vi "HFRR ADV v017 new software.vi"() -> ()   [LabVIEW 2025] (continued)
            n2021 = String To Path(string=w2022) -> (path=w2030:path)
            n2022 = String To Path(string=w2021) -> (path=w2029:path)
            n2023 = String To Path(string=w2020) -> (path=w2028:path)
            n2024 = case shown="True" w2019 {
              tunnel: [w2035 w2036] -> w2023
              frame False {
                n2025 = local read "string1"() -> (w2035:string)
              }
              frame True {
                n2026 = local read "String Indicator 4"() -> (w2036:string)
              }
            }
            n2027 = Open/Create/Replace File "Open File"(file path (use dialog)=w2030) -> (refnum out=w2026:refnum<file>)  [unwired: 5 in, 2 out]
            n2028 = Open/Create/Replace File "Open File"(file path (use dialog)=w2029) -> (refnum out=w2025:refnum<file>)  [unwired: 5 in, 2 out]
            n2029 = Open/Create/Replace File "Open File"(file path (use dialog)=w2028) -> (refnum out=w2024:refnum<file>)  [unwired: 5 in, 2 out]
            n2030 = while {
              tunnel: w2026 -> [w2048]
              i -> [w2044]
              stop <- w2043 continue-if-true
              (unwired) TRUE ("line mode (F)")
              n2031 = Read from Text File "Read File"(file (use dialog)=w2048) -> (text=w2045:string)  [unwired: 3 in, 3 out]
              n2032 = local write "Numeric 11"(w2044) -> ()
              n2033 = String Length(string=w2045) -> (length=w2047:i32)
              n2034 = Greater?(x=w2047, y=1) -> (0:w2043:bool)
            }
            n2035 = while {
              tunnel: w2025 -> [w2054]
              i -> [w2050]
              stop <- w2049 continue-if-true
              (unwired) TRUE ("line mode (F)")
              n2036 = Read from Text File "Read File"(file (use dialog)=w2054) -> (text=w2051:string)  [unwired: 3 in, 3 out]
              n2037 = local write "Numeric 12"(w2050) -> ()
              n2038 = String Length(string=w2051) -> (length=w2053:i32)
              n2039 = Greater?(x=w2053, y=1) -> (0:w2049:bool)
            }
            n2040 = while {
              tunnel: w2024 -> [w2060]
              i -> [w2056]
              stop <- w2055 continue-if-true
              (unwired) TRUE ("line mode (F)")
              n2041 = Read from Text File "Read File"(file (use dialog)=w2060) -> (text=w2057:string)  [unwired: 3 in, 3 out]
              n2042 = local write "Numeric 13"(w2056) -> ()
              n2043 = String Length(string=w2057) -> (length=w2059:i32)
              n2044 = Greater?(x=w2059, y=1) -> (0:w2055:bool)
            }
            n2045 = String To Path(string=w2023) -> (path=w2031:path)
            n2046 = Open/Create/Replace File "Open File"(file path (use dialog)=w2031) -> (refnum out=w2027:refnum<file>)  [unwired: 5 in, 2 out]
            n2047 = while {
              tunnel: w2027 -> [w2042]
              i -> [w2038]
              stop <- w2037 continue-if-true
              (unwired) TRUE ("line mode (F)")
              n2048 = Read from Text File "Read File"(file (use dialog)=w2042) -> (text=w2039:string)  [unwired: 3 in, 3 out]
              n2049 = local write "Numeric 8"(w2038) -> ()
              n2050 = String Length(string=w2039) -> (length=w2041:i32)
              n2051 = Greater?(x=w2041, y=1) -> (0:w2037:bool)
            }
          }
          frame #1 {
            w2212 = FALSE ("ACTUAL   MERGE")
            # "Sample Temp"
            # "ECR"
            # "COF"
            # "Time\nCOF\nFF\nTemp"
            n2052 = case shown="True" w2085 {
              tunnel: [w2232 w2233] -> w2086
              frame False {
                n2053 = local read "string1"() -> (w2232:string)
              }
              frame True {
                n2054 = local read "String Indicator 4"() -> (w2233:string)
              }
            }
            n2055 = local read "string1 3"() -> (w2130:string)
            n2056 = String To Path(string=w2086) -> (path=w2217:path)
            n2057 = String To Path(string=w2130) -> (path=w2228:path)
            n2058 = local read "Numeric 12"() -> (w2214:i32)
            n2059 = local read "Numeric 8"() -> (w2216:i32)
            n2060 = local read "string1 2"() -> (w2131:string)
            n2061 = local read "string1 4"() -> (w2129:string)
            n2062 = Open/Create/Replace File "Open File"(file path (use dialog)=w2217) -> (refnum out=w2231:refnum<file>, error out=w2230:errorcluster)  [unwired: 5 in, 1 out]
            n2063 = Open/Create/Replace File "Open File"(file path (use dialog)=w2228) -> (refnum out=w2224:refnum<file>, error out=w2225:errorcluster)  [unwired: 5 in, 1 out]
            n2064 = for {
              N: w2216 -> [_]
              tunnel: w2231 -> [w2379]
              tunnel: w2230 -> [w2378]
              tunnel: [w2368] -> w2143 mode=indexing
              tunnel: [w2366] -> w2200 mode=indexing
              tunnel: [w2367] -> w2195 mode=indexing
              tunnel: w2212 -> [_]
              tunnel: [w2360] -> w2197 mode=indexing
              tunnel: [w2356] -> w2166 mode=indexing
              tunnel: [w2352] -> w2141 mode=indexing
              tunnel: [w2348] -> w2122 mode=indexing
              tunnel: [w2343] -> w2082 mode=indexing
              (unwired) TRUE ("line mode (F)")
              # "freq"
              # "Stroke"
              # "Time"
              # "CoF"
              # "Humidity"
              # "Temp"
              # "Air Temp"
              # "ECR"
              n2065 = Read from Text File "Read File"(file (use dialog)=w2379, error in=w2378) -> (text=w2344:string)  [unwired: 2 in, 3 out]
              n2066 = local write "String 6"(w2344) -> ()
              n2067 = String Subset(string=w2344, offset (0)=0, length (rest)=14 ("length (rest)")) -> (substring=w2372:string)
              n2068 = String Subset(string=w2344, offset (0)=35, length (rest)=9 ("length (rest)")) -> (substring=w2369:string)
              n2069 = String Subset(string=w2344, offset (0)=15, length (rest)=9 ("length (rest)")) -> (substring=w2375:string)
              n2070 = Fract/Exp String To Number(string=w2372) -> (number=w2368:dbl)  [unwired: 3 in, 1 out]
              n2071 = Fract/Exp String To Number(string=w2369) -> (number=w2367:dbl)  [unwired: 3 in, 1 out]
              n2072 = Fract/Exp String To Number(string=w2375) -> (number=w2366:dbl)  [unwired: 3 in, 1 out]
              n2073 = String Subset(string=w2344, offset (0)=85, length (rest)=9 ("length (rest)")) -> (substring=w2345:string)
              n2074 = String Subset(string=w2344, offset (0)=25, length (rest)=9 ("length (rest)")) -> (substring=w2351:string)
              n2075 = String Subset(string=w2344, offset (0)=55, length (rest)=9 ("length (rest)")) -> (substring=w2353:string)
              n2076 = String Subset(string=w2344, offset (0)=45, length (rest)=9 ("length (rest)")) -> (substring=w2359:string)
              n2077 = String Subset(string=w2344, offset (0)=65, length (rest)=9 ("length (rest)")) -> (substring=w2365:string)
              n2078 = Fract/Exp String To Number(string=w2351) -> (number=w2348:dbl)  [unwired: 3 in, 1 out]
              n2079 = Fract/Exp String To Number(string=w2345) -> (number=w2343:dbl)  [unwired: 3 in, 1 out]
              n2080 = Fract/Exp String To Number(string=w2353) -> (number=w2352:dbl)  [unwired: 3 in, 1 out]
              n2081 = Fract/Exp String To Number(string=w2359) -> (number=w2356:dbl)  [unwired: 3 in, 1 out]
              n2082 = Fract/Exp String To Number(string=w2365) -> (number=w2362:dbl)  [unwired: 3 in, 1 out]
              n2083 = Add(x=w2362, y=0.0) -> (x+y=w2360:dbl)
            }
            n2084 = for {
              N: w2214 -> [_]
              tunnel: w2225 -> [w2305]
              tunnel: w2224 -> [w2304]
              tunnel: [w2294] -> w2183 mode=indexing
              tunnel: [w2292] -> w2181 mode=indexing
              tunnel: [w2293] -> w2177 mode=indexing
              tunnel: w2212 -> [_]
              tunnel: [w2286] -> w2179 mode=indexing
              tunnel: [w2282] -> w2161 mode=indexing
              tunnel: [w2278] -> w2137 mode=indexing
              tunnel: [w2275] -> w2118 mode=indexing
              tunnel: [w2271] -> w2077 mode=indexing
              (unwired) 9 ("length (rest)")
              (unwired) 9 ("length (rest)")
              (unwired) TRUE ("line mode (F)")
              n2085 = Read from Text File "Read File"(file (use dialog)=w2304, error in=w2305) -> (text=w2272:string)  [unwired: 2 in, 3 out]
              n2086 = local write "String 8"(w2272) -> ()
              n2087 = String Subset(string=w2272, offset (0)=85) -> (substring=w2274:string)  [unwired: 1 in]
              n2088 = String Subset(string=w2272, offset (0)=35, length (rest)=9 ("length (rest)")) -> (substring=w2295:string)
              n2089 = String Subset(string=w2272, offset (0)=55, length (rest)=9 ("length (rest)")) -> (substring=w2280:string)
              n2090 = String Subset(string=w2272, offset (0)=25) -> (substring=w2276:string)  [unwired: 1 in]
              n2091 = String Subset(string=w2272, offset (0)=15, length (rest)=9 ("length (rest)")) -> (substring=w2301:string)
              n2092 = String Subset(string=w2272, offset (0)=0, length (rest)=14 ("length (rest)")) -> (substring=w2298:string)
              n2093 = String Subset(string=w2272, offset (0)=45, length (rest)=9 ("length (rest)")) -> (substring=w2285:string)
              n2094 = String Subset(string=w2272, offset (0)=65, length (rest)=9 ("length (rest)")) -> (substring=w2291:string)
              n2095 = Fract/Exp String To Number(string=w2274) -> (number=w2271:dbl)  [unwired: 3 in, 1 out]
              n2096 = Fract/Exp String To Number(string=w2295) -> (number=w2293:dbl)  [unwired: 3 in, 1 out]
              n2097 = Fract/Exp String To Number(string=w2280) -> (number=w2278:dbl)  [unwired: 3 in, 1 out]
              n2098 = Fract/Exp String To Number(string=w2276) -> (number=w2275:dbl)  [unwired: 3 in, 1 out]
              n2099 = Fract/Exp String To Number(string=w2301) -> (number=w2292:dbl)  [unwired: 3 in, 1 out]
              n2100 = Fract/Exp String To Number(string=w2298) -> (number=w2294:dbl)  [unwired: 3 in, 1 out]
              n2101 = Fract/Exp String To Number(string=w2285) -> (number=w2282:dbl)  [unwired: 3 in, 1 out]
              n2102 = Fract/Exp String To Number(string=w2291) -> (number=w2288:dbl)  [unwired: 3 in, 1 out]
              n2103 = Add(x=w2288, y=0.0) -> (x+y=w2286:dbl)
            }
            n2104 = String To Path(string=w2131) -> (path=w2229:path)
            n2105 = String To Path(string=w2129) -> (path=w2223:path)
            n2106 = local read "Numeric 11"() -> (w2213:i32)
            n2107 = local read "Numeric 13"() -> (w2215:i32)
            n2108 = Open/Create/Replace File "Open File"(file path (use dialog)=w2229) -> (refnum out=w2227:refnum<file>, error out=w2226:errorcluster)  [unwired: 5 in, 1 out]
            n2109 = Open/Create/Replace File "Open File"(file path (use dialog)=w2223) -> (refnum out=w2222:refnum<file>, error out=w2221:errorcluster)  [unwired: 5 in, 1 out]
            n2110 = for {
              N: w2213 -> [_]
              tunnel: w2227 -> [w2342]
              tunnel: w2226 -> [w2341]
              tunnel: [w2331] -> w2193 mode=indexing
              tunnel: [w2329] -> w2191 mode=indexing
              tunnel: [w2330] -> w2186 mode=indexing
              tunnel: w2212 -> [_]
              tunnel: [w2323] -> w2188 mode=indexing
              tunnel: [w2319] -> w2164 mode=indexing
              tunnel: [w2315] -> w2139 mode=indexing
              tunnel: [w2311] -> w2120 mode=indexing
              tunnel: [w2306] -> w2078 mode=indexing
              (unwired) TRUE ("line mode (F)")
              n2111 = Read from Text File "Read File"(file (use dialog)=w2342, error in=w2341) -> (text=w2307:string)  [unwired: 2 in, 3 out]
              n2112 = local write "String 7"(w2307) -> ()
              n2113 = String Subset(string=w2307, offset (0)=85, length (rest)=9 ("length (rest)")) -> (substring=w2310:string)
              n2114 = String Subset(string=w2307, offset (0)=35, length (rest)=9 ("length (rest)")) -> (substring=w2332:string)
              n2115 = String Subset(string=w2307, offset (0)=55, length (rest)=9 ("length (rest)")) -> (substring=w2318:string)
              n2116 = String Subset(string=w2307, offset (0)=25, length (rest)=9 ("length (rest)")) -> (substring=w2312:string)
              n2117 = String Subset(string=w2307, offset (0)=45, length (rest)=9 ("length (rest)")) -> (substring=w2320:string)
              n2118 = String Subset(string=w2307, offset (0)=0, length (rest)=14 ("length (rest)")) -> (substring=w2335:string)
              n2119 = String Subset(string=w2307, offset (0)=15, length (rest)=9 ("length (rest)")) -> (substring=w2338:string)
              n2120 = String Subset(string=w2307, offset (0)=65, length (rest)=9 ("length (rest)")) -> (substring=w2324:string)
              n2121 = Fract/Exp String To Number(string=w2310) -> (number=w2306:dbl)  [unwired: 3 in, 1 out]
              n2122 = Fract/Exp String To Number(string=w2332) -> (number=w2330:dbl)  [unwired: 3 in, 1 out]
              n2123 = Fract/Exp String To Number(string=w2318) -> (number=w2315:dbl)  [unwired: 3 in, 1 out]
              n2124 = Fract/Exp String To Number(string=w2312) -> (number=w2311:dbl)  [unwired: 3 in, 1 out]
              n2125 = Fract/Exp String To Number(string=w2320) -> (number=w2319:dbl)  [unwired: 3 in, 1 out]
              n2126 = Fract/Exp String To Number(string=w2335) -> (number=w2331:dbl)  [unwired: 3 in, 1 out]
              n2127 = Fract/Exp String To Number(string=w2338) -> (number=w2329:dbl)  [unwired: 3 in, 1 out]
              n2128 = Fract/Exp String To Number(string=w2324) -> (number=w2327:dbl)  [unwired: 3 in, 1 out]
              n2129 = Add(x=w2327, y=0.0) -> (x+y=w2323:dbl)
            }
            n2130 = for {
              N: w2215 -> [_]
              tunnel: w2222 -> [w2270]
              tunnel: w2221 -> [w2269]
              tunnel: [w2259] -> w2175 mode=indexing
              tunnel: [w2258] -> w2168 mode=indexing
              tunnel: w2212 -> [_]
              tunnel: [w2247] -> w2173 mode=indexing
              tunnel: [w2252] -> w2170 mode=indexing
              tunnel: [w2248] -> w2160 mode=indexing
              tunnel: [w2243] -> w2135 mode=indexing
              tunnel: [w2239] -> w2116 mode=indexing
              tunnel: [w2234] -> w2076 mode=indexing
              (unwired) 1.0 ("x")
              (unwired) TRUE ("line mode (F)")
              n2131 = Read from Text File "Read File"(file (use dialog)=w2270, error in=w2269) -> (text=w2235:string)  [unwired: 2 in, 3 out]
              n2132 = local write "String 12"(w2235) -> ()
              n2133 = String Subset(string=w2235, offset (0)=85, length (rest)=9 ("length (rest)")) -> (substring=w2237:string)
              n2134 = String Subset(string=w2235, offset (0)=35, length (rest)=9 ("length (rest)")) -> (substring=w2260:string)
              n2135 = String Subset(string=w2235, offset (0)=55, length (rest)=9 ("length (rest)")) -> (substring=w2245:string)
              n2136 = String Subset(string=w2235, offset (0)=25, length (rest)=9 ("length (rest)")) -> (substring=w2241:string)
              n2137 = String Subset(string=w2235, offset (0)=45, length (rest)=9 ("length (rest)")) -> (substring=w2250:string)
              n2138 = String Subset(string=w2235, offset (0)=15, length (rest)=9 ("length (rest)")) -> (substring=w2266:string)
              n2139 = String Subset(string=w2235, offset (0)=0, length (rest)=14 ("length (rest)")) -> (substring=w2263:string)
              n2140 = String Subset(string=w2235, offset (0)=65, length (rest)=9 ("length (rest)")) -> (substring=w2253:string)
              n2141 = Fract/Exp String To Number(string=w2237) -> (number=w2234:dbl)  [unwired: 3 in, 1 out]
              n2142 = Fract/Exp String To Number(string=w2260) -> (number=w2258:dbl)  [unwired: 3 in, 1 out]
              n2143 = Fract/Exp String To Number(string=w2245) -> (number=w2243:dbl)  [unwired: 3 in, 1 out]
              n2144 = Fract/Exp String To Number(string=w2241) -> (number=w2239:dbl)  [unwired: 3 in, 1 out]
              n2145 = Fract/Exp String To Number(string=w2250) -> (number=w2248:dbl)  [unwired: 3 in, 1 out]
              n2146 = Fract/Exp String To Number(string=w2266) -> (number=w2247:dbl)  [unwired: 3 in, 1 out]
              n2147 = Fract/Exp String To Number(string=w2263) -> (number=w2259:dbl)  [unwired: 3 in, 1 out]
              n2148 = Fract/Exp String To Number(string=w2253) -> (number=w2256:dbl)  [unwired: 3 in, 1 out]
              n2149 = Add(x=w2256, y=0.0) -> (x+y=w2252:dbl)
            }
            n2150 = Delete From Array(array=w2118, index=0) -> (array with subset deleted=w2091:dbl[])  [unwired: 1 in, 1 out]
            n2151 = Delete From Array(array=w2181, index=0) -> (array with subset deleted=w2154:dbl[])  [unwired: 1 in, 1 out]
            n2152 = Delete From Array(array=w2161, index=0) -> (array with subset deleted=w2149:dbl[])  [unwired: 1 in, 1 out]
            n2153 = Delete From Array(array=w2179, index=0) -> (array with subset deleted=w2180:dbl[])  [unwired: 1 in, 1 out]
            n2154 = call-poly <vilib>:"Mean.vi"("X"=w2091) -> ("mean"=→"КОФ2 4":dbl)  [unwired: 1 out]
            n2155 = call-poly <vilib>:"Mean.vi"("X"=w2154) -> ("mean"=→"КОФ3":dbl)  [unwired: 1 out]
            n2156 = call-poly <vilib>:"Mean.vi"("X"=w2149) -> ("mean"=→"CP3":dbl)  [unwired: 1 out]
            n2157 = Delete From Array(array=w2143, index=0) -> (array with subset deleted=w2070:dbl[])  [unwired: 1 in, 1 out]
            n2158 = Delete From Array(array=w2082, index=0) -> (array with subset deleted=w2069:dbl[])  [unwired: 1 in, 1 out]
            n2159 = Delete From Array(array=w2122, index=0) -> (array with subset deleted=w2093:dbl[])  [unwired: 1 in, 1 out]
            n2160 = Delete From Array(array=w2200, index=0) -> (array with subset deleted=w2155:dbl[])  [unwired: 1 in, 1 out]
            n2161 = Delete From Array(array=w2166, index=0) -> (array with subset deleted=w2151:dbl[])  [unwired: 1 in, 1 out]
            "array w/ subset deleted" <- w2151
            n2162 = Delete From Array(array=w2197, index=0) -> (array with subset deleted=w2198:dbl[])  [unwired: 1 in, 1 out]
            n2163 = call-poly <vilib>:"Mean.vi"("X"=w2093) -> ("mean"=→"КОФ2 2":dbl)  [unwired: 1 out]
            n2164 = call-poly <vilib>:"Mean.vi"("X"=w2155) -> ("mean"=→"КОФ1":dbl)  [unwired: 1 out]
            n2165 = Bundle "Bundle"(w2070, w2069) -> (w2075:cluster{dbl[], dbl[]})  [unwired: 1 in]
            n2166 = Bundle "Bundle"(w2070, w2198) -> (w2062:cluster{dbl[], dbl[]})  [unwired: 1 in]
            n2167 = Delete From Array(array=w2077, index=0) -> (array with subset deleted=w2065:dbl[])  [unwired: 1 in, 1 out]
            n2168 = Delete From Array(array=w2078, index=0) -> (array with subset deleted=w2067:dbl[])  [unwired: 1 in, 1 out]
            n2169 = Delete From Array(array=w2188, index=0) -> (array with subset deleted=w2189:dbl[])  [unwired: 1 in, 1 out]
            n2170 = Delete From Array(array=w2076, index=0) -> (array with subset deleted=w2063:dbl[])  [unwired: 1 in, 1 out]
            n2171 = Delete From Array(array=w2170, index=0) -> (array with subset deleted=w2171:dbl[])  [unwired: 1 in, 1 out]
            n2172 = Delete From Array(array=w2195, index=0) -> (array with subset deleted=w2101:dbl[])  [unwired: 1 in, 1 out]
            n2173 = Delete From Array(array=w2141, index=0) -> (array with subset deleted=w2097:dbl[])  [unwired: 1 in, 1 out]
            n2174 = Delete From Array(array=w2177, index=0) -> (array with subset deleted=w2099:dbl[])  [unwired: 1 in, 1 out]
            n2175 = Delete From Array(array=w2137, index=0) -> (array with subset deleted=w2095:dbl[])  [unwired: 1 in, 1 out]
            n2176 = Delete From Array(array=w2186, index=0) -> (array with subset deleted=w2100:dbl[])  [unwired: 1 in, 1 out]
            n2177 = Delete From Array(array=w2139, index=0) -> (array with subset deleted=w2096:dbl[])  [unwired: 1 in, 1 out]
            n2178 = Delete From Array(array=w2120, index=0) -> (array with subset deleted=w2092:dbl[])  [unwired: 1 in, 1 out]
            n2179 = Delete From Array(array=w2164, index=0) -> (array with subset deleted=w2150:dbl[])  [unwired: 1 in, 1 out]
            n2180 = Delete From Array(array=w2191, index=0) -> (array with subset deleted=w2152:dbl[])  [unwired: 1 in, 1 out]
            n2181 = Delete From Array(array=w2168, index=0) -> (array with subset deleted=w2098:dbl[])  [unwired: 1 in, 1 out]
            n2182 = Delete From Array(array=w2135, index=0) -> (array with subset deleted=w2094:dbl[])  [unwired: 1 in, 1 out]
            n2183 = Delete From Array(array=w2116, index=0) -> (array with subset deleted=w2090:dbl[])  [unwired: 1 in, 1 out]
            n2184 = Delete From Array(array=w2160, index=0) -> (array with subset deleted=w2148:dbl[])  [unwired: 1 in, 1 out]
            n2185 = Delete From Array(array=w2173, index=0) -> (array with subset deleted=w2153:dbl[])  [unwired: 1 in, 1 out]
            n2186 = Delete From Array(array=w2183, index=0) -> (array with subset deleted=w2066:dbl[])  [unwired: 1 in, 1 out]
            n2187 = Delete From Array(array=w2193, index=0) -> (array with subset deleted=w2068:dbl[])  [unwired: 1 in, 1 out]
            n2188 = Delete From Array(array=w2175, index=0) -> (array with subset deleted=w2064:dbl[])  [unwired: 1 in, 1 out]
            n2189 = Bundle "Bundle"(w2070, w2101) -> (w2088:cluster{dbl[], dbl[]})  [unwired: 1 in]
            n2190 = Bundle "Bundle"(w2070, w2155) -> (w2089:cluster{dbl[], dbl[]})  [unwired: 1 in]
            n2191 = Bundle "Bundle"(w2101, w2097) -> (w2103:cluster{dbl[], dbl[]})  [unwired: 1 in]
            n2192 = Bundle "Bundle"(w2066, w2065) -> (w2073:cluster{dbl[], dbl[]})  [unwired: 1 in]
            n2193 = Bundle "Bundle"(w2099, w2095) -> (w2105:cluster{dbl[], dbl[]})  [unwired: 1 in]
            n2194 = Bundle "Bundle"(w2066, w2099) -> (w2209:cluster{dbl[], dbl[]})  [unwired: 1 in]
            n2195 = Bundle "Bundle"(w2066, w2095) -> (w2133:cluster{dbl[], dbl[]})  [unwired: 1 in]
            n2196 = Bundle "Bundle"(w2066, w2154) -> (w2219:cluster{dbl[], dbl[]})  [unwired: 1 in]
            n2197 = Bundle "Bundle"(w2066, w2149) -> (w2157:cluster{dbl[], dbl[]})  [unwired: 1 in]
            n2198 = Bundle "Bundle"(w2066, w2180) -> (w2204:cluster{dbl[], dbl[]})  [unwired: 1 in]
            n2199 = Bundle "Bundle"(w2100, w2096) -> (w2104:cluster{dbl[], dbl[]})  [unwired: 1 in]
            n2200 = Bundle "Bundle"(w2068, w2067) -> (w2074:cluster{dbl[], dbl[]})  [unwired: 1 in]
            n2201 = Bundle "Bundle"(w2068, w2100) -> (w2211:cluster{dbl[], dbl[]})  [unwired: 1 in]
            n2202 = Bundle "Bundle"(w2068, w2096) -> (w2134:cluster{dbl[], dbl[]})  [unwired: 1 in]
            n2203 = Bundle "Bundle"(w2068, w2150) -> (w2158:cluster{dbl[], dbl[]})  [unwired: 1 in]
            n2204 = Bundle "Bundle"(w2068, w2152) -> (w2220:cluster{dbl[], dbl[]})  [unwired: 1 in]
            n2205 = Bundle "Bundle"(w2068, w2189) -> (w2202:cluster{dbl[], dbl[]})  [unwired: 1 in]
            n2206 = Bundle "Bundle"(w2098, w2094) -> (w2106:cluster{dbl[], dbl[]})  [unwired: 1 in]
            n2207 = Bundle "Bundle"(w2064, w2063) -> (w2072:cluster{dbl[], dbl[]})  [unwired: 1 in]
            n2208 = Bundle "Bundle"(w2064, w2098) -> (w2210:cluster{dbl[], dbl[]})  [unwired: 1 in]
            n2209 = Bundle "Bundle"(w2064, w2094) -> (w2132:cluster{dbl[], dbl[]})  [unwired: 1 in]
            n2210 = Bundle "Bundle"(w2064, w2148) -> (w2156:cluster{dbl[], dbl[]})  [unwired: 1 in]
            n2211 = Bundle "Bundle"(w2064, w2153) -> (w2218:cluster{dbl[], dbl[]})  [unwired: 1 in]
            n2212 = Bundle "Bundle"(w2064, w2171) -> (w2203:cluster{dbl[], dbl[]})  [unwired: 1 in]
            n2213 = call-poly <vilib>:"Mean.vi"("X"=w2151) -> ("mean"=→"CP1":dbl)  [unwired: 1 out]
            n2214 = call-poly <vilib>:"Mean.vi"("X"=w2092) -> ("mean"=→"КОФ2 3":dbl)  [unwired: 1 out]
            n2215 = call-poly <vilib>:"Mean.vi"("X"=w2150) -> ("mean"=→"CP2":dbl)  [unwired: 1 out]
            n2216 = call-poly <vilib>:"Mean.vi"("X"=w2152) -> ("mean"=→"КОФ2":dbl)  [unwired: 1 out]
            n2217 = call-poly <vilib>:"Mean.vi"("X"=w2090) -> ("mean"=→"КОФ2 5":dbl)  [unwired: 1 out]
            n2218 = call-poly <vilib>:"Mean.vi"("X"=w2148) -> ("mean"=→"CP4":dbl)  [unwired: 1 out]
            n2219 = call-poly <vilib>:"Mean.vi"("X"=w2153) -> ("mean"=→"КОФ4":dbl)  [unwired: 1 out]
            n2220 = Bundle "Bundle"(w2070, w2097) -> (w2061:cluster{dbl[], dbl[]})  [unwired: 1 in]
            n2221 = Bundle "Bundle"(w2070, w2151) -> (w2084:cluster{dbl[], dbl[]})  [unwired: 1 in]
            n2222 = Build Array "Build Array"(w2061, w2084) -> (w2087:cluster{dbl[], dbl[]}[])
            "XY Graph 17" <- w2087
            n2223 = Build Array "Build Array"(w2075, w2074, w2073, w2072) -> (→"Frequency ( Hz )":cluster{dbl[], dbl[]}[])
            n2224 = Build Array "Build Array"(w2103, w2104, w2105, w2106) -> (→"Air Temp ( °C ) vs Humidity ( % RH )":cluster{dbl[], dbl[]}[])
            n2225 = Build Array "Build Array"(w2088, w2211, w2209, w2210) -> (→"Air Temperature  ( °C )":cluster{dbl[], dbl[]}[])
            n2226 = Build Array "Build Array"(w2061, w2134, w2133, w2132) -> (→"Humidity ( %RH )":cluster{dbl[], dbl[]}[])
            n2227 = Build Array "Build Array"(w2089, w2220, w2219, w2218) -> (→"Coefficient Of Friction":cluster{dbl[], dbl[]}[])
            n2228 = Build Array "Build Array"(w2084, w2158, w2157, w2156) -> (→"Sample Temperature ( °C )":cluster{dbl[], dbl[]}[])
            n2229 = Build Array "Build Array"(w2062, w2202, w2204, w2203) -> (→"XY Graph 13":cluster{dbl[], dbl[]}[])
            n2230 = Bundle "Bundle"(w2070, w2093) -> (w2115:cluster{dbl[], dbl[]})  [unwired: 1 in]
            n2231 = Bundle "Bundle"(w2066, w2091) -> (w2113:cluster{dbl[], dbl[]})  [unwired: 1 in]
            n2232 = Bundle "Bundle"(w2068, w2092) -> (w2114:cluster{dbl[], dbl[]})  [unwired: 1 in]
            n2233 = Bundle "Bundle"(w2064, w2090) -> (w2112:cluster{dbl[], dbl[]})  [unwired: 1 in]
            n2234 = Build Array "Build Array"(w2115, w2114, w2113, w2112) -> (→"Stroke ( mm )":cluster{dbl[], dbl[]}[])
            n2235 = local write "XY Graph 16"(w2087) -> ()
          }
          frame #2 {
          }
          frame #3 {
            n2236 = local write "Numeric 8"(0 ("Numeric 8")) -> ()
            n2237 = local write "Numeric 11"(0 ("Numeric 11")) -> ()
            n2238 = local write "Numeric 12"(0 ("Numeric 12")) -> ()
            n2239 = local write "Numeric 13"(0 ("Numeric 13")) -> ()
            n2240 = property on="OPEN" class="Bool (strict)"("Visible"=TRUE) -> ()  [unwired: 2 in, 2 out]
            n2241 = local read "String Control 2"() -> (w2387:string)
            n2242 = local read "String Control 4"() -> (w2386:string)
            n2243 = local read "String Control 6"() -> (w2385:string)
            n2244 = local read "String Control 8"() -> (w2384:string)
            n2245 = Match Pattern(string=w2387, regular expression="Samples / cycle :- ") -> (after substring=w2401:string)  [unwired: 1 in, 3 out]
            n2246 = Match Pattern(string=w2387, regular expression="Frequency :- ") -> (after substring=w2420:string)  [unwired: 1 in, 3 out]
            n2247 = Match Pattern(string=w2386, regular expression="Samples / cycle :- ") -> (after substring=w2397:string)  [unwired: 1 in, 3 out]
            n2248 = Match Pattern(string=w2386, regular expression="Frequency :- ") -> (after substring=w2415:string)  [unwired: 1 in, 3 out]
            n2249 = Match Pattern(string=w2385, regular expression="Samples / cycle :- ") -> (after substring=w2393:string)  [unwired: 1 in, 3 out]
            n2250 = Match Pattern(string=w2385, regular expression="Frequency :- ") -> (after substring=w2410:string)  [unwired: 1 in, 3 out]
            n2251 = Match Pattern(string=w2384, regular expression="Samples / cycle :- ") -> (after substring=w2389:string)  [unwired: 1 in, 3 out]
            n2252 = Match Pattern(string=w2384, regular expression="Frequency :- ") -> (after substring=w2405:string)  [unwired: 1 in, 3 out]
            n2253 = String Subset(string=w2401, length (rest)=6 ("length (rest)")) -> (substring=w2403:string)  [unwired: 1 in]
            n2254 = String Subset(string=w2420, length (rest)=9 ("length (rest)")) -> (substring=w2422:string)  [unwired: 1 in]
            n2255 = String Subset(string=w2397, length (rest)=6 ("length (rest)")) -> (substring=w2399:string)  [unwired: 1 in]
            n2256 = String Subset(string=w2415, length (rest)=9 ("length (rest)")) -> (substring=w2417:string)  [unwired: 1 in]
            n2257 = String Subset(string=w2393, length (rest)=6 ("length (rest)")) -> (substring=w2395:string)  [unwired: 1 in]
            n2258 = String Subset(string=w2410, length (rest)=9 ("length (rest)")) -> (substring=w2412:string)  [unwired: 1 in]
            n2259 = String Subset(string=w2389, length (rest)=6 ("length (rest)")) -> (substring=w2391:string)  [unwired: 1 in]
            n2260 = String Subset(string=w2405, length (rest)=9 ("length (rest)")) -> (substring=w2407:string)  [unwired: 1 in]
            n2261 = Fract/Exp String To Number(string=w2403) -> (number=w2383:dbl)  [unwired: 3 in, 1 out]
            n2262 = Fract/Exp String To Number(string=w2422) -> (number=w2423:dbl)  [unwired: 3 in, 1 out]
            n2263 = Fract/Exp String To Number(string=w2399) -> (number=w2382:dbl)  [unwired: 3 in, 1 out]
            n2264 = Fract/Exp String To Number(string=w2417) -> (number=w2418:dbl)  [unwired: 3 in, 1 out]
            n2265 = Fract/Exp String To Number(string=w2395) -> (number=w2381:dbl)  [unwired: 3 in, 1 out]
            n2266 = Fract/Exp String To Number(string=w2412) -> (number=w2413:dbl)  [unwired: 3 in, 1 out]
            n2267 = Fract/Exp String To Number(string=w2391) -> (number=w2380:dbl)  [unwired: 3 in, 1 out]
            n2268 = Fract/Exp String To Number(string=w2407) -> (number=w2408:dbl)  [unwired: 3 in, 1 out]
            n2269 = local write "sample1"(w2383) -> ()
            n2270 = local write "freq1"(w2423) -> ()
            n2271 = local write "sample2"(w2382) -> ()
            n2272 = local write "freq2"(w2418) -> ()
            n2273 = local write "sample3"(w2381) -> ()
            n2274 = local write "freq3"(w2413) -> ()
            n2275 = local write "sample4"(w2380) -> ()
            n2276 = local write "freq 4"(w2408) -> ()
          }
        }
      }
    }
    n2277 = case shown="True" w1872 {
      selector: w1872 -> [_ w2000]
      frame False {
      }
      frame True {
        n2278 = Not(x=w2000) -> (.not. x?=w1996:bool)
        n2279 = local write "service 3"(w1996) -> ()
        n2280 = local write "OPEN 6"(w1996) -> ()
        n2281 = call <vilib>:"System Exec.vi"("wait until completion? (T)"=TRUE, "command line"="C:\\LAB-IQ\\Scar View.exe") -> ("error out"=→"error out 5":errorcluster)  [unwired: 6 in, 3 out]
      }
    }
    n2282 = case shown="\"Acquire\", Default" w1883 {
      frame "Acquire", Default {
        w2896 = 0.2 ("y")
        w2901 = 1.0 ("y")
        w2902 = 0.8 ("y")
        # "Elapsed time\ncof\nstroke\nAir temp\nTemp\nHumidity"
        n2283 = disable-structure shown="Disabled" {
          frame Disabled {
            n2284 = local read "Flag"() -> (w2919:dbl)
            n2285 = local read "RUN"() -> (w2916:bool)
            n2286 = Not(x=w2916) -> (.not. x?=w2915:bool)
            n2287 = Equal?(x=w2919, y=10.0) -> (x = y?=w2917:bool)
            n2288 = And(x=w2917, y=w2915) -> (x .and. y?=w2914:bool)
            n2289 = case shown="True" w2914 {
              frame False {
              }
              frame True {
                w2920 = FALSE ("Heater Button")
                n2290 = local write "Humidity"(w2920) -> ()
                n2291 = local write "Heater Button"(w2920) -> ()
              }
            }
          }
          frame Enabled {
          }
        }
        n2292 = disable-structure shown="Disabled" {
          frame Disabled {
            n2293 = case shown="True" {
              selector: _ -> [_ _]
              frame False {
              }
              frame True {
                w3011 = TRUE ("Heater")
                n2294 = local write "Humidity"(w3011) -> ()
                n2295 = local write "Heater Button"(w3011) -> ()
                n2296 = local read "TEST STANDARD"() -> (w3014:T3)
                n2297 = local read "TEST STANDARD"() -> (w3009:T3)
                n2298 = Equal?(x=w3014, y=enum16{"ASTM D6079", "ISO 12156", "Custom"}."ISO 12156" ("Test Standard")) -> (x = y?=w3012:bool)
                n2299 = Equal?(x=w3009, y=enum16{"ASTM D6079", "ISO 12156", "Custom"}."ASTM D6079" ("Test Standard")) -> (x = y?=w3008:bool)
                n2300 = case shown="True" w3012 {
                  frame False {
                  }
                  frame True {
                    n2301 = local write "Heater"(TRUE ("Heater")) -> ()
                    n2302 = local write "airtempflg"(FALSE ("airtempflg")) -> ()
                  }
                }
                n2303 = case shown="True" w3008 {
                  frame False {
                  }
                  frame True {
                    n2304 = local write "Heater"(FALSE ("Heater")) -> ()
                    n2305 = local write "airtempflg"(TRUE ("airtempflg")) -> ()
                  }
                }
              }
            }
          }
          frame Enabled {
          }
        }
        n2306 = stacked-sequence {
          frame #0 {
            n2307 = case shown="True" "RST FF" {
              frame False {
              }
              frame True {
                w3077 = 0.0 ("X Scale.Range:Maximum")
                n2308 = property on="Frictional Force ( N )" class="WFChart (strict)"("XScale.Maximum"=600.0 ("X Scale.Range:Maximum"), "XScale.Minimum"=w3077, "YScale.Maximum"=10.0 ("Y Scale.Range:Maximum"), "YScale.Minimum"=w3077) -> ()  [unwired: 2 in, 2 out]
              }
            }
          }
          frame #1 {
            n2309 = case shown="True" "RST TEMP" {
              frame False {
              }
              frame True {
                n2310 = property on="Temperature ( Deg C )" class="WFChart (strict)"("XScale.Minimum"=0.0 ("X Scale.Range:Minimum"), "XScale.Maximum"=600.0 ("X Scale.Range:Maximum"), "YScale.Minimum"=0.0 ("Y Scale.Range:Minimum"), "YScale.Maximum"=100.0 ("Y Scale.Range:Maximum")) -> ()  [unwired: 2 in, 2 out]
              }
            }
          }
          frame #2 {
            n2311 = case shown="True" "RSTCOF" {
              frame False {
              }
              frame True {
                n2312 = property on="Coefficient of Friction" class="WFChart (strict)"("XScale.Minimum"=0.0 ("X Scale.Range:Minimum"), "XScale.Maximum"=600.0 ("X Scale.Range:Maximum"), "YScale.Maximum"=1.0 ("X Scale.Range:Minimum"), "YScale.Minimum"=0.0 ("X Scale.Range:Minimum")) -> ()  [unwired: 2 in, 2 out]
              }
            }
          }
          frame #3 {
            n2313 = case shown="True" "RSTCOF 2" {
              frame False {
              }
              frame True {
                (unwired) 100.0 ("Y Scale.Range:Maximum")
                (unwired) 0.0 ("Y Scale.Range:Minimum")
                (unwired) 600.0 ("X Scale.Range:Maximum")
                (unwired) 0.0 ("X Scale.Range:Minimum")
              }
            }
          }
          frame #4 {
            n2314 = case shown="True" "RSTCOF 3" {
              frame False {
              }
              frame True {
                n2315 = property on="Electrical Contact Resistance ( % )" class="WFChart (strict)"("XScale.Minimum"=0.0 ("X Scale.Range:Minimum"), "XScale.Maximum"=600.0 ("X Scale.Range:Maximum"), "YScale.Minimum"=0.0 ("Y Scale.Range:Minimum"), "YScale.Maximum"=100.0 ("Y Scale.Range:Maximum")) -> ()  [unwired: 2 in, 2 out]
              }
            }
          }
        }
        n2316 = disable-structure shown="Disabled" {
          frame Disabled {
            n2317 = case shown="True" {
              selector: _ -> [_ _]
              frame False {
              }
              frame True {
                n2318 = local read "zflag 2"() -> (w2978:dbl)
                n2319 = local read "yflag"() -> (w2980:dbl)
                n2320 = Equal?(x=w2980, y=2.0 ("tflag")) -> (x = y?=w2982:bool)
                n2321 = Equal?(x=w2978, y=3.0 ("tflag")) -> (x = y?=w2981:bool)
                n2322 = And(x=w2982, y=w2981) -> (x .and. y?=w2976:bool)
                n2323 = case shown="True" w2976 {
                  frame False {
                  }
                  frame True {
                    w3007 = 0.0 ("zflag")
                    n2324 = local write "zflag"(w3007) -> ()
                    n2325 = local write "zflag 2"(w3007) -> ()
                    n2326 = Delete(path (use dialog)=path "C:/LAB-IQ-NXT/WO 2449 TT.sig" ("file path (dialog if empty)")) -> (deleted path=w3006:path)  [unwired: 4 in, 2 out]
                    n2327 = Delete(path (use dialog)=path "C:/LAB-IQ-NXT/WO 2449 TRH.sig" ("file path (dialog if empty)")) -> (deleted path=w3001:path)  [unwired: 4 in, 2 out]
                    n2328 = local read "SEN.RUN HRS"() -> (w2993:dbl)
                    n2329 = local read "SENSOR TIME"() -> (w2991:dbl)
                    n2330 = call <vilib>:"compatOverwrite.vi"("overwrite (F)"=TRUE) -> ("overwrite?"=w2983:T30)
                    n2331 = call <vilib>:"compatOverwrite.vi"("overwrite (F)"=TRUE) -> ("overwrite?"=w2987:T30)
                    n2332 = local read "Total No. of Tests"() -> (w2994:dbl)
                    n2333 = Add(x=w2991, y=w2993) -> (x+y=w2992:dbl)
                    "SEN.RUN HRS" <- w2992
                    n2334 = Open/Create/Replace File(file path (use dialog)=w3006, operation (0:open)=w2983) -> (refnum out=w2984:refnum<file>, error out=w2985:errorcluster)  [unwired: 4 in, 1 out]
                    n2335 = Open/Create/Replace File(file path (use dialog)=w3001, operation (0:open)=w2987) -> (refnum out=w2988:refnum<file>, error out=w2989:errorcluster)  [unwired: 4 in, 1 out]
                    n2336 = Deny Access(4:w2985, 6:T28."deny none" ("deny mode (2)"), 7:w2984) -> (3:w3005:refnum<file>)  [unwired: 1 out]
                    n2337 = Deny Access(4:w2989, 6:T28."deny none" ("deny mode (2)"), 7:w2988) -> (3:w2997:refnum<file>)  [unwired: 1 out]
                    n2338 = Number To Decimal String(number=w2994) -> (decimal integer string=w3002:string)  [unwired: 1 in]
                    n2339 = Number To Decimal String(number=w2992) -> (decimal integer string=w2998:string)  [unwired: 1 in]
                    n2340 = Write to Binary File(file (use dialog)=w3005, data=w3002, 5:FALSE ("prepend array or string size? (T)")) -> ()  [unwired: 3 in, 3 out]
                    n2341 = Write to Binary File(file (use dialog)=w2997, data=w2998, 5:FALSE ("prepend array or string size? (T)")) -> ()  [unwired: 3 in, 3 out]
                  }
                }
              }
            }
          }
          frame Enabled {
          }
        }
        n2342 = local read "RUN"() -> (w2905:bool)
        n2343 = local read "run replace"() -> (w2909:bool)
        n2344 = local read "run replace"() -> (w2908:bool)
        n2345 = case shown="True" w2905 {
          frame False {
            n2346 = local write "run replace"(FALSE ("run replace")) -> ()
          }
          frame True {
            "run replace" <- TRUE ("run replace")
          }
        }
        n2347 = local read "RUN"() -> (w2913:bool)
        n2348 = local read "Set Temp"() -> (w2875:dbl)
        n2349 = local read "SetTemp"() -> (w2877:dbl)
        n2350 = case shown="False" w2913 {
          tunnel: [FALSE ("TEST RUNNING") TRUE ("TEST RUNNING")] -> w2912
          frame False {
            w3096 = 0.0 ("Flag")
            n2351 = local write "Elapsed time"(0.0 ("elapsedtime")) -> ()
            n2352 = local write "Time Remaining"(w3096) -> ()
            n2353 = local write "Flag"(w3096) -> ()
            n2354 = local write "Remaining Time"(w3096) -> ()
          }
          frame True {
            n2355 = local write "Flag"(10.0 ("Flag")) -> ()
          }
        }
        n2356 = case shown="False" w2909 {
          frame False {
            n2357 = local read "zflag"() -> (→"zflag 2":dbl)
            n2358 = local write "yflag"(2.0 ("tflag")) -> ()
            n2359 = local write "FLAG 4"(0.0 ("FLAG")) -> ()
          }
          frame True {
            n2360 = local write "yflag"(1.0 ("tflag")) -> ()
            n2361 = local write "zflag"(3.0 ("zflag")) -> ()
          }
        }
        n2362 = local read "acq 2"() -> (w2907:bool)
        n2363 = local read "AIR TEMP"() -> (w2870:dbl)
        n2364 = local read "Amb temp"() -> (w2874:dbl)
        n2365 = case shown="True" "Save & Continue" {
          frame False {
          }
          frame True {
            "acq 2" <- TRUE ("acq 2")
          }
        }
        n2366 = local read "Set Rh"() -> (w2876:dbl)
        n2367 = Add(x=w2877, y=w2902) -> (x+y=w2903:dbl)
        n2368 = Subtract(x=w2877, y=w2902) -> (x-y=w2904:dbl)
        n2369 = Add(x=w2875, y=w2896) -> (x+y=w2897:dbl)
        n2370 = Subtract(x=w2875, y=w2896) -> (x-y=w2898:dbl)
        n2371 = And(x=w2907, y=w2908) -> (x .and. y?=w2906:bool)
        n2372 = Greater Or Equal?(x=w2870, y=15.0) -> (x >= y?=w2871:bool)
        "powstat" <- w2871
        n2373 = local read "Humidity ( %RH )"() -> (w2873:dbl)
        n2374 = case shown="True" "Save & Continue" {
          frame False {
          }
          frame True {
            n2375 = while {
              tunnel: "0123456789abcdefghijklmnopqrstuvwxyzABCDEFGHIJKLMNOPQRSTUVWXYZ" ("string 2") -> [w3067]
              shift-right: [w3065] -> w3060
              shift-left: "" -> [w3064]
              i -> [w3074]
              stop <- w3073 stop-if-true
              n2376 = Random Number (0-1)() -> (number: 0 to 1=w3068:dbl)
              n2377 = Multiply(x=w3068, y=62.0) -> (x*y=w3070:dbl)
              n2378 = Decrement(x="Length") -> (x-1=w3063:i16)
              n2379 = To Word Integer(number=w3070) -> (16bit integer=w3071:i16)
              n2380 = String Subset(string=w3067, offset (0)=w3071, length (rest)=1 ("length (rest)")) -> (substring=w3066:string)
              n2381 = Greater Or Equal?(x=w3074, y=w3063) -> (x >= y?=w3073:bool)
              n2382 = Concatenate Strings(w3066, w3064) -> (w3065:string)
            }
            n2383 = local write "UUID"(w3060) -> ()
          }
        }
        n2384 = In Range and Coerce(upper limit=w2903, x=w2874, lower limit=w2904) -> (In Range?=w2893:bool)  [unwired: 1 out]
        n2385 = Add(x=w2876, y=w2901) -> (x+y=w2900:dbl)
        n2386 = Subtract(x=w2876, y=w2901) -> (x-y=w2899:dbl)
        n2387 = local read "TEMP"() -> (w2872:dbl)
        n2388 = case shown="True" "Save & Continue" {
          frame False {
          }
          frame True {
            n2389 = local read "Operator ID"() -> (w3391:string)
            n2390 = local read "FILE"() -> (w3397:string)
            n2391 = String Length(string=w3397) -> (length=w3395:i32)
            n2392 = String Length(string=w3391) -> (length=w3392:i32)
            n2393 = Greater?(x=w3395, y=0) -> (0:w3394:bool)
            n2394 = Greater?(x=w3392, y=0) -> (0:w3390:bool)
            n2395 = And(x=w3394, y=w3390) -> (x .and. y?=w3389:bool)
            n2396 = case shown="True" w3389 {
              frame False {
                n2397 = stacked-sequence {
                  frame #0 {
                    n2398 = One Button Dialog(message="Please Enter a File Name and Operator ID to save data !", button name ("OK")="Ok") -> ()  [unwired: 1 out]
                  }
                  frame #1 {
                    n2399 = local write "Save & Continue"(FALSE ("OK Button")) -> ()
                  }
                }
                n2400 = local write "Save & Continue"(FALSE ("OK Button")) -> ()
              }
              frame True {
                n2401 = stacked-sequence {
                  frame #0 {
                    n2402 = local read "FILE"() -> (w3403:string)
                    n2403 = call "file check.vi"("file name in"=w3403) -> ("file name out"=w3402:string)  [unwired: 9 in, 1 out]
                    n2404 = call <vilib>:"Application Directory.vi"() -> ("Application Directory"=w3413:path)
                    n2405 = Build Path(base path=w3413, name or relative path="data") -> (appended path=w3412:path)
                    n2406 = call <vilib>:"Trim Whitespace.vi"("string"=w3402) -> ("trimmed string"=w3410:string)  [unwired: 1 in]
                    n2407 = call <vilib>:"Trim Whitespace.vi"("string"=w3402) -> ("trimmed string"=w3411:string)  [unwired: 1 in]
                    n2408 = List Folder(path=w3412) -> (folder names=w3408:string[])  [unwired: 3 in, 3 out]
                    n2409 = Match Pattern(string=w3410, regular expression="_(") -> (before substring=w3407:string)  [unwired: 1 in, 3 out]
                    n2410 = for {
                      tunnel: w3408 -> [w3422] mode=indexing
                      tunnel: w3407 -> [w3420]
                      shift-right: [w3418] -> w3405
                      shift-left: bool[] [] -> [w3419]
                      n2411 = Match Pattern(string=w3422, regular expression="_(") -> (before substring=w3421:string)  [unwired: 1 in, 3 out]
                      n2412 = Equal?(x=w3421, y=w3420) -> (x = y?=w3417:bool)
                      n2413 = case shown="True" w3417 {
                        tunnel: w3417 -> [_ w3425]
                        tunnel: w3419 -> [w3424 w3427]
                        tunnel: [w3424 w3426] -> w3418
                        frame False {
                        }
                        frame True {
                          n2414 = Insert Into Array(array=w3427, new element=w3425) -> (w3426:bool[])  [unwired: 1 in]
                        }
                      }
                    }
                    n2415 = Equal?(x=w3408, y=w3407) -> (x = y?=w3416:bool[])
                    n2416 = Or Array Elements(Boolean array=w3416) -> (logical OR=w3415:bool)
                    n2417 = Array Size(array=w3405) -> (size(s)=w3404:i32)
                    n2418 = case shown="True" w3415 {
                      tunnel: w3411 -> [_ w3435]
                      tunnel: w3404 -> [_ w3428]
                      frame False {
                      }
                      frame True {
                        n2419 = Number To Decimal String(number=w3428) -> (decimal integer string=w3431:string)  [unwired: 1 in]
                        n2420 = Search/Split String(string=w3435, search string/char (-)="_(" ("regular expression")) -> (substring before match=w3433:string)  [unwired: 1 in, 2 out]
                        n2421 = Concatenate Strings(w3433, "_(" ("regular expression"), w3431, ")" ("regular expression")) -> (w3429:string)
                        n2422 = local write "FILE"(w3429) -> ()
                      }
                    }
                  }
                  frame #1 {
                    w3437 = 0.0
                    w3450 = cluster{"y":dbl, dbl, "y":dbl}[] [] ("History Data")
                    w3451 = FALSE ("Heater Button")
                    (unwired) ")!" ("string")
                    (unwired) ")" ("string")
                    w3449 = dbl[] [] ("History Data")
                    w3455 = "\r"
                    # "C:\\WinDucom\\Data\\"
                    # "C:\\LAB-IQ-NXT\\data"
                    n2423 = local write "Humidity ( %RH )"(w3437) -> ()
                    n2424 = local write "Frequency ( Hz )"(w3437) -> ()
                    n2425 = local write "Stroke 3"(w3437) -> ()
                    n2426 = local write "speedop"(0.0 ("PIDclk 2")) -> ()
                    n2427 = local write "Set Temp 2"(65.0 ("Set Temp 2")) -> ()
                    n2428 = local write "AIR TEMP"(w3437) -> ()
                    n2429 = local write "clk"(0.0 ("clk")) -> ()
                    n2430 = local write "Stroke 4"(w3437) -> ()
                    n2431 = local write "COF 2"(w3437) -> ()
                    n2432 = local write "TEMP"(w3437) -> ()
                    n2433 = local write "ecr 3"(w3437) -> ()
                    n2434 = local write "FF 3"(w3437) -> ()
                    n2435 = local write "FF 2"(w3437) -> ()
                    n2436 = property on="Humidity ( %RH )" class="WFChart (strict)"("History Data"=w3449) -> ()  [unwired: 2 in, 2 out]
                    n2437 = property on="Coefficient of Friction" class="WFChart (strict)"("History Data"=w3449) -> ()  [unwired: 2 in, 2 out]
                    n2438 = property on="Coefficient of Friction" class="WFChart (strict)"("History Data"=w3449) -> ()  [unwired: 2 in, 2 out]
                    n2439 = property on="Frictional Force ( N )" class="WFChart (strict)"("History Data"=w3449) -> ()  [unwired: 2 in, 2 out]
                    n2440 = property on="Electrical Contact Resistance ( % )" class="WFChart (strict)"("History Data"=w3449) -> ()  [unwired: 2 in, 2 out]
                    n2441 = property on="Electrical Contact Resistance ( % )" class="WFChart (strict)"("History Data"=w3449) -> ()  [unwired: 2 in, 2 out]
                    n2442 = property on="Temperature ( Deg C )" class="WFChart (strict)"("History Data"=w3449) -> ()  [unwired: 2 in, 2 out]
                    n2443 = property on="Frictional Force ( N )" class="WFChart (strict)"("History Data"=w3449) -> ()  [unwired: 2 in, 2 out]
                    n2444 = property on="Coefficient of Friction" class="WFChart (strict)"("History Data"=w3449) -> ()  [unwired: 2 in, 2 out]
                    n2445 = property on="Frictional Force ( N )" class="WFChart (strict)"("History Data"=w3449) -> ()  [unwired: 2 in, 2 out]
                    n2446 = property on="Electrical Contact Resistance ( % )" class="WFChart (strict)"("History Data"=w3449) -> ()  [unwired: 2 in, 2 out]
                    n2447 = property on="Temperature ( Deg C )" class="WFChart (strict)"("History Data"=w3449) -> ()  [unwired: 2 in, 2 out]
                    n2448 = property on="Humidity ( %RH )" class="WFChart (strict)"("History Data"=w3449) -> ()  [unwired: 2 in, 2 out]
                    n2449 = property on="Stroke ( mm )" class="WFChart (strict)"("History Data"=w3450) -> ()  [unwired: 2 in, 2 out]
                    n2450 = property on="Stroke ( mm )" class="WFChart (strict)"("History Data"=w3450) -> ()  [unwired: 2 in, 2 out]
                    n2451 = local write "Humidity"(w3451) -> ()
                    n2452 = local write "Heater Button"(w3451) -> ()
                    n2453 = local read "FILE"() -> (w3445:string)
                    n2454 = disable-structure shown="Enabled" {
                      disable-tunnel: [w3490 _] -> w3436
                      frame Enabled {
                        n2455 = local read "NORMAL LOAD"() -> (w3490:dbl)
                      }
                      frame Disabled {
                      }
                    }
                    n2456 = call "file check.vi"("file name in"=w3445) -> ("error out"=w3448:errorcluster, "file name out"=w3442:string)  [unwired: 9 in]
                    n2457 = call "FILE PATH CREATION.vi"("error in"=w3448, "FILE NAME :"=w3442) -> ("FILE OUT"=w3441:path)  [unwired: 8 in, 1 out]
                    n2458 = Concatenate Strings(w3442, ".dgf" ("Substring")) -> (w3447:string)
                    n2459 = Concatenate Strings(w3442, ".duf" ("Substring")) -> (w3443:string)
                    n2460 = Multiply(x=w3436, y=1.0) -> (x*y=w3469:dbl)
                    n2461 = Build Path(base path=w3441, name or relative path=w3447) -> (appended path=w3440:path)
                    n2462 = Build Path(base path=w3441, name or relative path=w3443) -> (appended path=w3439:path)
                    n2463 = Number To Fractional String(number=w3469, width (-)=i16 5, precision (6)=i16 2) -> (F-format string=w3477:string)  [unwired: 1 in]
                    n2464 = local read "Fuel Discription :"() -> (w3465:string)
                    n2465 = local read "Batch Ref Num :"() -> (w3453:string)
                    n2466 = Get Date/Time String(date format (0)=enum16{"short", "long", "abbreviated"}."short") -> (date string=w3488:string, time string=w3485:string)  [unwired: 2 in]
                    n2467 = local read "Remarks :"() -> (w3464:string)
                    n2468 = Concatenate Strings("Load :- " ("Substring"), w3477, " grams ," ("Substring")) -> (w3476:string)
                    n2469 = local read "String 41"() -> (w3456:string)
                    n2470 = Concatenate Strings(w3465) -> (w3466:string)
                    n2471 = Concatenate Strings(w3453) -> (w3452:string)
                    n2472 = Concatenate Strings("tested by") -> (w3460:string)
                    n2473 = Concatenate Strings("(" ("Substring"), w3488, ")" ("Substring"), w3485) -> (w3458:string)
                    "concatenated string" <- w3458
                    n2474 = Concatenate Strings(w3464, "," ("string")) -> (w3463:string)
                    n2475 = Concatenate Strings("  TIME;      COF;       STROKE;     AIR TEMP;  TEMP;  HUMIDITY;  ECR; PID-OUT; FREQUENCY" ("Substring"), "\r") -> (w3472:string)
                    n2476 = Concatenate Strings(w3456, w3455, "Fuel Discription :-" ("Substring"), w3466, w3455, w3476, w3455, "Batch Ref Num :-" ("Substring"), w3452, w3455, " Remarks :- " ("Substring"), w3463, w3455, " Date :- " ("Substring"), w3458, w3455, "Tested By :-" ("Substring"), w3460) -> (w3470:string)
                    "REMARKS" <- w3470
                    n2477 = call <vilib>:"Write Characters To File.vi"("append to file? (new file:F)"=FALSE, "character string"=w3472, "file path (dialog if empty)"=w3440) -> ()  [unwired: 2 in, 1 out]
                    n2478 = call <vilib>:"Write Characters To File.vi"("append to file? (new file:F)"=FALSE, "character string"=w3470, "file path (dialog if empty)"=w3439) -> ()  [unwired: 2 in, 1 out]
                  }
                  frame #2 {
                    n2479 = local write "Cycles elapsed"(0 ("Cycles elapsed")) -> ()
                    n2480 = local write "cyclecount"(0 ("cyclecount")) -> ()
                    n2481 = local write "Save & Continue"(FALSE ("OK")) -> ()
                    n2482 = local write "autostrtflg"(TRUE ("autostrtflg")) -> ()
                    n2483 = local write "Save"(FALSE ("Save")) -> ()
                    n2484 = Get Date/Time In Seconds() -> (seconds since 1Jan1904=w3495:timestamp)
                    n2485 = To Double Precision Float(number=w3495) -> (double precision float=w3494:dbl)
                    n2486 = local write "acq timer"(w3494) -> ()
                    n2487 = One Button Dialog(message="Please ensure sample is mounted properly and machine is ready in all aspects for testing !", button name ("OK")="Ok") -> ()  [unwired: 1 out]
                  }
                  frame #3 {
                    n2488 = stacked-sequence {
                      frame #0 {
                        n2489 = local write "Main Dashboard Buttons"(T1."Dashboard" ("Main Dashboard Buttons")) -> ()
                        n2490 = local write "Main Tab"(T2."Acquire" ("Main Tab")) -> ()
                      }
                      frame #1 {
                        n2491 = local write "EVENT LOG"("" ("EVENT LOG")) -> ()
                      }
                      frame #2 {
                        n2492 = Wait (ms)(milliseconds to wait=u32 50) -> ()  [unwired: 1 out]
                      }
                      frame #3 {
                        n2493 = disable-structure shown="Disabled" {
                          frame Disabled {
                            n2494 = local read "EVENT LOG"() -> (w3507:string)
                            n2495 = call "Event Log.vi"("Content"="Test Details", "EVENT LOG"=w3507) -> ("EVENT LOG"=w3506:string)  [unwired: 8 in, 1 out]
                            n2496 = local write "EVENT LOG"(w3506) -> ()
                          }
                          frame Enabled {
                          }
                        }
                      }
                      frame #4 {
                        n2497 = Wait (ms)(milliseconds to wait=u32 50) -> ()  [unwired: 1 out]
                      }
                      frame #5 {
                        n2498 = local read "FILE"() -> (w3509:string)
                        n2499 = Concatenate Strings("File Name :" ("Content"), w3509) -> (w3510:string)
                        n2500 = local read "EVENT LOG"() -> (w3513:string)
                        n2501 = call "Event Log.vi"("Content"=w3510, "EVENT LOG"=w3513) -> ("EVENT LOG"=w3512:string)  [unwired: 8 in, 1 out]
                        n2502 = local write "EVENT LOG"(w3512) -> ()
                      }
                      frame #6 {
                        n2503 = Wait (ms)(milliseconds to wait=u32 50) -> ()  [unwired: 1 out]
                      }
                      frame #7 {
                        n2504 = local read "Batch Ref Num :"() -> (w3515:string)
                        n2505 = Concatenate Strings("Batch Ref No :" ("Content"), w3515) -> (w3516:string)
                        n2506 = local read "EVENT LOG"() -> (w3519:string)
                        n2507 = call "Event Log.vi"("Content"=w3516, "EVENT LOG"=w3519) -> ("EVENT LOG"=w3518:string)  [unwired: 8 in, 1 out]
                        n2508 = local write "EVENT LOG"(w3518) -> ()
                      }
                      frame #8 {
                        n2509 = Wait (ms)(milliseconds to wait=u32 50) -> ()  [unwired: 1 out]
                      }
                      frame #9 {
                        n2510 = local read "tested by"() -> (w3521:string)
                        n2511 = Concatenate Strings("Tested By :" ("Content"), w3521) -> (w3522:string)
                        n2512 = local read "EVENT LOG"() -> (w3525:string)
                        n2513 = call "Event Log.vi"("Content"=w3522, "EVENT LOG"=w3525) -> ("EVENT LOG"=w3524:string)  [unwired: 8 in, 1 out]
                        n2514 = local write "EVENT LOG"(w3524) -> ()
                      }
                      frame #10 {
                        n2515 = Wait (ms)(milliseconds to wait=u32 50) -> ()  [unwired: 1 out]
                      }
                      frame #11 {
                        n2516 = local read "TEST STANDARD"() -> (w3528:T3)
                        n2517 = case shown="\"ASTM D6079\", Default" w3528 {
                          tunnel: ["ASTM D6079" "ISO 12156" "CEC F-096-A-06" "Custom"] -> w3527
                          frame "ASTM D6079", Default {
                          }
                          frame "ISO 12156" {
                          }
                          frame "CEC F-096-A-06" {
                          }
                          frame "Custom" {
                          }
                        }
                        n2518 = Concatenate Strings("Test Standard :" ("Content"), w3527) -> (w3529:string)
                        n2519 = local read "EVENT LOG"() -> (w3532:string)
                        n2520 = call "Event Log.vi"("Content"=w3529, "EVENT LOG"=w3532) -> ("EVENT LOG"=w3531:string)  [unwired: 8 in, 1 out]
                        n2521 = local write "EVENT LOG"(w3531) -> ()
                      }
                      frame #12 {
                        n2522 = Wait (ms)(milliseconds to wait=u32 50) -> ()  [unwired: 1 out]
                      }
                      frame #13 {
                        n2523 = local read "Fuel Discription :"() -> (w3538:string)
                        n2524 = Concatenate Strings("Fuel Description :" ("Content"), w3538) -> (w3539:string)
                        n2525 = local read "EVENT LOG"() -> (w3542:string)
                        n2526 = call "Event Log.vi"("Content"=w3539, "EVENT LOG"=w3542) -> ("EVENT LOG"=w3541:string)  [unwired: 8 in, 1 out]
                        n2527 = local write "EVENT LOG"(w3541) -> ()
                      }
                      frame #14 {
                        n2528 = Wait (ms)(milliseconds to wait=u32 50) -> ()  [unwired: 1 out]
                      }
                      frame #15 {
                        n2529 = local read "Remarks :"() -> (w3544:string)
                        n2530 = Concatenate Strings("Remarks :" ("Content"), w3544) -> (w3545:string)
                        n2531 = local read "EVENT LOG"() -> (w3548:string)
                        n2532 = call "Event Log.vi"("Content"=w3545, "EVENT LOG"=w3548) -> ("EVENT LOG"=w3547:string)  [unwired: 8 in, 1 out]
                        n2533 = local write "EVENT LOG"(w3547) -> ()
                      }
                      frame #16 {
                        n2534 = Wait (ms)(milliseconds to wait=u32 50) -> ()  [unwired: 1 out]
                      }
                      frame #17 {
                        n2535 = local read "Operator ID"() -> (w3550:string)
                        n2536 = Concatenate Strings("Operator ID :" ("Content"), w3550) -> (w3552:string)
                        n2537 = local read "EVENT LOG"() -> (w3554:string)
                        n2538 = call "Event Log.vi"("Content"=w3552, "EVENT LOG"=w3554) -> ("EVENT LOG"=w3553:string)  [unwired: 8 in, 1 out]
                        n2539 = local write "EVENT LOG"(w3553) -> ()
                      }
                      frame #18 {
                        n2540 = Wait (ms)(milliseconds to wait=u32 50) -> ()  [unwired: 1 out]
                      }
                      frame #19 {
                        n2541 = disable-structure shown="Disabled" {
                          frame Disabled {
                            n2542 = local read "EVENT LOG"() -> (w3558:string)
                            n2543 = call "Event Log.vi"("Content"="Test Parameter", "EVENT LOG"=w3558) -> ("EVENT LOG"=w3557:string)  [unwired: 8 in, 1 out]
                            n2544 = local write "EVENT LOG"(w3557) -> ()
                          }
                          frame Enabled {
                          }
                        }
                      }
                      frame #20 {
                        n2545 = Wait (ms)(milliseconds to wait=u32 50) -> ()  [unwired: 1 out]
                      }
                      frame #21 {
                        n2546 = local read "Set Hz"() -> (w3562:dbl)
